vi "Lab Panel V5.22.1.vi"() -> ()   [LabVIEW 2013] (continued)
            n171 = local write "Error USB #0"(w189) -> ()
            n172 = local write "Reset Error"(w189) -> ()
            n173 = local write "Error USB #1"(w189) -> ()
            n174 = local write "Error USB #2"(w189) -> ()
          }
        }
        frame #8 {
          # "get initial temperature values"
          n175 = stacked-sequence {
            frame #0 {
              w196 = T12 {"T1 Live"=20.0, "T1 Neut"=20.0, "T2 Live"=20.0, "T2 Neut"=20.0, "ID"=6.0, "ER"=10.0} ("LAB01 TEMP")
              n176 = local write "LAB deg C"(w196) -> ()
              n177 = global write "Global display 4.vi" "LAB deg C"(w196) -> ()
              n178 = local write "OFF amps"(1.5) -> ()
              n179 = local write "ON amps"(20.0) -> ()
              n180 = local write "VOLTS"(250.0) -> ()
              n181 = local write "PF"(0.5) -> ()
            }
            frame #1 {
              w241 = TRUE
              n182 = local read "Simulate"() -> (w203:bool)
              n183 = local write "Panel #"(0) -> ()
              n184 = case shown="True" w203 {
                frame False {
                }
                frame True {
                  w243 = 20
                  n185 = local write "Ambient Volts"(2.92) -> ()
                  n186 = global write "Global display 3.vi" "Ref deg C"(w243) -> ()
                  n187 = local write "Ref deg C"(w243) -> ()
                }
              }
              n188 = call "sub vi - GET ALL TEMP v7.vi"("LA01-EN"=w241, "simulate"=w203, "LA02-EN"=w241, "LA03-EN"=w241, "LA04-EN"=w241, "LA05-EN"=w241, "Gen Cal Value"=1) -> ("ID"=w202:T24, "LA01 TEMP"=w239:T25, "LA02 TEMP"=w232:T25, "LA03 TEMP"=w225:T25, "LA04 TEMP"=w218:T25, "LA05 TEMP"=w211:T25)  [unwired: 2 in, 1 out]
              n189 = local write "LAB05 TEMP"(w211) -> ()
              n190 = local write "LAB04 TEMP"(w218) -> ()
              n191 = Unbundle(w225) -> ("T1"=w222:dbl, "T2"=w221:dbl, "T3"=w220:dbl, "T4"=w219:dbl)  [unwired: 2 out]
              n192 = Unbundle(w239) -> ("T1"=w237:dbl, "T2"=w236:dbl, "T3"=w235:dbl, "T4"=w234:dbl)  [unwired: 2 out]
              n193 = Unbundle(w232) -> ("T1"=w229:dbl, "T2"=w228:dbl, "T3"=w227:dbl, "T4"=w226:dbl)  [unwired: 2 out]
              n194 = Unbundle(w218) -> ("T1"=w216:dbl, "T2"=w215:dbl, "T3"=w214:dbl, "T4"=w213:dbl)  [unwired: 2 out]
              n195 = Unbundle(w211) -> ("T1"=w209:dbl, "T2"=w208:dbl, "T3"=w207:dbl, "T4"=w206:dbl)  [unwired: 2 out]
              n196 = local write "LAB01 TEMP"(w239) -> ()
              n197 = local write "LAB02 TEMP"(w232) -> ()
              n198 = local write "LAB03 TEMP"(w225) -> ()
              n199 = Unbundle(w202) -> ("id1"=→"LAB01-TP":bool, "id2"=→"LAB02-TP":bool, "id3"=→"LAB03-TP":bool, "id4"=→"LAB04-TP":bool, "id5"=→"LAB05-TP":bool)
              n200 = local read "TEMP LA05"() -> (w210:T9)
              n201 = local read "TEMP LA04"() -> (w217:T9)
              n202 = local read "TEMP LA02"() -> (w231:T9)
              n203 = local read "TEMP LA03"() -> (w224:T9)
              n204 = local read "TEMP LA01"() -> (w238:T9)
              n205 = Bundle(cluster=w224, "TL-1"=w222, "TN-1"=w221, "TL-2"=w220, "TN-2"=w219) -> (w223:T9)  [unwired: 4 in]
              n206 = Bundle(cluster=w238, "TL-1"=w237, "TN-1"=w236, "TL-2"=w235, "TN-2"=w234) -> (w233:T9)  [unwired: 4 in]
              n207 = Bundle(cluster=w231, "TL-1"=w229, "TN-1"=w228, "TL-2"=w227, "TN-2"=w226) -> (w230:T9)  [unwired: 4 in]
              n208 = Bundle(cluster=w217, "TL-1"=w216, "TN-1"=w215, "TL-2"=w214, "TN-2"=w213) -> (w212:T9)  [unwired: 4 in]
              n209 = Bundle(cluster=w210, "TL-1"=w209, "TN-1"=w208, "TL-2"=w207, "TN-2"=w206) -> (w205:T9)  [unwired: 4 in]
              n210 = local write "TEMP LA03"(w223) -> ()
              n211 = local write "TEMP LA01"(w233) -> ()
              n212 = local write "TEMP LA02"(w230) -> ()
              n213 = local write "TEMP LA05"(w205) -> ()
              n214 = local write "TEMP LA04"(w212) -> ()
            }
            frame #2 {
              w252 = 0
              n215 = local read "LAB01 TEMP"() -> (w254:T12)
              n216 = local read "SIG LAB01-2"() -> (w249:T2)
              n217 = Unbundle By Name(w254) -> ("T1 Live"=w247:dbl, "T1 Neut"=w246:dbl, "T2 Live"=w245:dbl, "T2 Neut"=w244:dbl)  [unwired: 2 out]
              n218 = local read "SIG LAB01-1"() -> (w251:T2)
              n219 = local read "TEMP LA01"() -> (w255:T9)
              n220 = Bundle By Name(cluster=w255, "TL-1"=w247, "TN-1"=w246, "TL-2"=w245, "TN-2"=w244, "TL -1COUNT"=w252, "TN-1 COUNT"=w252, "TL-2 COUNT"=w252, "TN-2 COUNT"=w252) -> (w253:T9)
              n221 = Bundle(cluster=w251, "Tmp Live"=w247, "Tmp Neut"=w246) -> (w250:T2)  [unwired: 3 in]
              n222 = Bundle(cluster=w249, "Tmp Live"=w245, "Tmp Neut"=w244) -> (w248:T2)  [unwired: 3 in]
              n223 = local write "SIG LAB01-2"(w248) -> ()
              n224 = local write "SIG LAB01-1"(w250) -> ()
              n225 = local write "TEMP LA01"(w253) -> ()
            }
            frame #3 {
              w264 = 0
              n226 = local read "LAB02 TEMP"() -> (w266:T12)
              n227 = Unbundle By Name(w266) -> ("T1 Live"=w259:dbl, "T1 Neut"=w258:dbl, "T2 Live"=w257:dbl, "T2 Neut"=w256:dbl)  [unwired: 2 out]
              n228 = local read "SIG LAB02-1"() -> (w263:T2)
              n229 = local read "SIG LAB02-2"() -> (w262:T2)
              n230 = local read "TEMP LA02"() -> (w267:T9)
              n231 = Bundle By Name(cluster=w267, "TL-1"=w259, "TN-1"=w258, "TL-2"=w257, "TN-2"=w256, "TL -1COUNT"=w264, "TN-1 COUNT"=w264, "TL-2 COUNT"=w264, "TN-2 COUNT"=w264) -> (w265:T9)
              n232 = Bundle(cluster=w262, "Tmp Live"=w257, "Tmp Neut"=w256) -> (w260:T2)  [unwired: 3 in]
              n233 = Bundle(cluster=w263, "Tmp Live"=w259, "Tmp Neut"=w258) -> (w261:T2)  [unwired: 3 in]
              n234 = local write "TEMP LA02"(w265) -> ()
              n235 = local write "SIG LAB02-1"(w261) -> ()
              n236 = local write "SIG LAB02-2"(w260) -> ()
            }
            frame #4 {
              w276 = 0
              n237 = local read "LAB03 TEMP"() -> (w278:T12)
              n238 = Unbundle By Name(w278) -> ("T1 Live"=w271:dbl, "T1 Neut"=w270:dbl, "T2 Live"=w269:dbl, "T2 Neut"=w268:dbl)  [unwired: 2 out]
              n239 = local read "SIG LAB03-1"() -> (w275:T2)
              n240 = local read "SIG LAB03-2"() -> (w274:T2)
              n241 = local read "TEMP LA03"() -> (w279:T9)
              n242 = Bundle By Name(cluster=w279, "TL-1"=w271, "TN-1"=w270, "TL-2"=w269, "TN-2"=w268, "TL -1COUNT"=w276, "TN-1 COUNT"=w276, "TL-2 COUNT"=w276, "TN-2 COUNT"=w276) -> (w277:T9)
              n243 = Bundle(cluster=w274, "Tmp Live"=w269, "Tmp Neut"=w268) -> (w272:T2)  [unwired: 3 in]
              n244 = Bundle(cluster=w275, "Tmp Live"=w271, "Tmp Neut"=w270) -> (w273:T2)  [unwired: 3 in]
              n245 = local write "TEMP LA03"(w277) -> ()
              n246 = local write "SIG LAB03-2"(w272) -> ()
              n247 = local write "SIG LAB03-1"(w273) -> ()
            }
            frame #5 {
              w288 = 0
              n248 = local read "LAB04 TEMP"() -> (w290:T12)
              n249 = Unbundle By Name(w290) -> ("T1 Live"=w283:dbl, "T1 Neut"=w282:dbl, "T2 Live"=w281:dbl, "T2 Neut"=w280:dbl)  [unwired: 2 out]
              n250 = local read "SIG LAB04-2"() -> (w286:T2)
              n251 = local read "SIG LAB04-1"() -> (w287:T2)
              n252 = local read "TEMP LA04"() -> (w291:T9)
              n253 = Bundle By Name(cluster=w291, "TL-1"=w283, "TN-1"=w282, "TL-2"=w281, "TN-2"=w280, "TL -1COUNT"=w288, "TN-1 COUNT"=w288, "TL-2 COUNT"=w288, "TN-2 COUNT"=w288) -> (w289:T9)
              n254 = Bundle(cluster=w286, "Tmp Live"=w281, "Tmp Neut"=w280) -> (w284:T2)  [unwired: 3 in]
              n255 = Bundle(cluster=w287, "Tmp Live"=w283, "Tmp Neut"=w282) -> (w285:T2)  [unwired: 3 in]
              n256 = local write "SIG LAB04-2"(w284) -> ()
              n257 = local write "TEMP LA04"(w289) -> ()
              n258 = local write "SIG LAB04-1"(w285) -> ()
            }
            frame #6 {
              w300 = 0
              n259 = local read "LAB05 TEMP"() -> (w302:T12)
              n260 = Unbundle By Name(w302) -> ("T1 Live"=w295:dbl, "T1 Neut"=w294:dbl, "T2 Live"=w293:dbl, "T2 Neut"=w292:dbl)  [unwired: 2 out]
              n261 = local read "SIG LAB05-2"() -> (w298:T2)
              n262 = local read "SIG LAB05-1"() -> (w299:T2)
              n263 = local read "TEMP LA05"() -> (w303:T9)
              n264 = Bundle By Name(cluster=w303, "TL-1"=w295, "TN-1"=w294, "TL-2"=w293, "TN-2"=w292, "TL -1COUNT"=w300, "TN-1 COUNT"=w300, "TL-2 COUNT"=w300, "TN-2 COUNT"=w300) -> (w301:T9)
              n265 = Bundle(cluster=w298, "Tmp Live"=w293, "Tmp Neut"=w292) -> (w296:T2)  [unwired: 3 in]
              n266 = Bundle(cluster=w299, "Tmp Live"=w295, "Tmp Neut"=w294) -> (w297:T2)  [unwired: 3 in]
              n267 = local write "SIG LAB05-2"(w296) -> ()
              n268 = local write "SIG LAB05-1"(w297) -> ()
              n269 = local write "TEMP LA05"(w301) -> ()
            }
          }
        }
        frame #9 {
          # "enable front panel, all settings done"
          n270 = property on="Tab Control 2" class="TabCtl (strict)"("DisabledEnum"=T16."Enabled" ("Disabled")) -> ()  [unwired: 2 in, 2 out]
          n271 = property on="Tab Control 2" class="TabCtl (strict)"("Value"=0) -> ()  [unwired: 2 in, 2 out]
        }
        frame #10 {
          n272 = property on="Tab Control 2" class="TabCtl (strict)"("Value"=0) -> ()  [unwired: 2 in, 2 out]
        }
      }
    }
    frame #2 {
      n273 = node-c288("loop  delay(mS)") -> (w309:T18)  [unwired: 3 in]
      n274 = timed-loop {
        timing: w309 -> [_]
        timing-out: [_] -> w308
        i -> [w335]
        stop <- w312 stop-if-true
        n275 = node-c288() -> ()  [unwired: 1 in, 1 out]
        n276 = local read "Resets Done"() -> (w314:dbl)
        n277 = Greater?(x=w314, y=30) -> (0:w310:bool)
        n278 = local read "SELECT LAB05-2"() -> (w315:T3)
        n279 = local read "SELECT LAB05-1"() -> (w316:T3)
        n280 = local read "SELECT LAB04-2"() -> (w317:T3)
        n281 = local read "SELECT LAB03-1"() -> (w320:T3)
        n282 = Or(x=w310, y="stop") -> (x .or. y?=w312:bool)
        n283 = local read "SELECT LAB02-2"() -> (w321:T3)
        n284 = local read "SELECT LAB01-1"() -> (w324:T3)
        n285 = local read "SELECT LAB03-2"() -> (w319:T3)
        n286 = local read "SELECT LAB01-2"() -> (w323:T3)
        n287 = local read "SELECT LAB04-1"() -> (w318:T3)
        n288 = local read "SELECT LAB02-1"() -> (w322:T3)
        n289 = local read "run lab03-2"() -> (w329:bool)
        n290 = local read "run lab04-1"() -> (w328:bool)
        n291 = local read "run lab05-1"() -> (w326:bool)
        n292 = local read "run lab04-2"() -> (w327:bool)
        n293 = local read "run lab05-2"() -> (w325:bool)
        n294 = local read "run lab03-1"() -> (w330:bool)
        n295 = local read "run lab02-2"() -> (w331:bool)
        n296 = local read "run lab02-1"() -> (w332:bool)
        n297 = local read "run lab01-1"() -> (w334:bool)
        n298 = local read "run lab01-2"() -> (w333:bool)
        n299 = global write "Global display 1.vi" "stop disp"(w312) -> ()
        n300 = stacked-sequence {
          seq-local: [_ w401 _ _ _ _ _ _ _ _ _ _ _ _ _ _ _ _ _ _ _ _ _] -> [_ _ _ _ _ w2502 _ _ _ _ _ _ _ _ _ _ _ _ _ _ _ _ _]
          seq-local: [_ w400 _ _ _ _ _ _ _ _ _ _ _ _ _ _ _ _ _ _ _ _ _] -> [_ _ _ _ _ w2501 _ _ _ _ _ _ _ _ _ _ _ _ _ _ _ _ _]
          seq-local: [_ w387 _ _ _ _ _ _ _ _ _ _ _ _ _ _ _ _ _ _ _ _ _] -> [_ _ _ _ _ w2500 _ _ _ _ _ _ _ _ _ _ _ _ _ _ _ _ _]
          seq-local: [_ w386 _ _ _ _ _ _ _ _ _ _ _ _ _ _ _ _ _ _ _ _ _] -> [_ _ _ _ _ w2499 _ _ _ _ _ _ _ _ _ _ _ _ _ _ _ _ _]
          seq-local: [_ w385 _ _ _ _ _ _ _ _ _ _ _ _ _ _ _ _ _ _ _ _ _] -> [_ _ _ _ _ w2498 _ _ _ _ _ _ _ _ _ _ _ _ _ _ _ _ _]
          seq-local: [_ w384 _ _ _ _ _ _ _ _ _ _ _ _ _ _ _ _ _ _ _ _ _] -> [_ _ _ _ _ w2497 _ _ _ _ _ _ _ _ _ _ _ _ _ _ _ _ _]
          seq-local: [_ w383 _ _ _ _ _ _ _ _ _ _ _ _ _ _ _ _ _ _ _ _ _] -> [_ _ _ _ _ w2496 _ _ _ _ _ _ _ _ _ _ _ _ _ _ _ _ _]
          seq-local: [_ w382 _ _ _ _ _ _ _ _ _ _ _ _ _ _ _ _ _ _ _ _ _] -> [_ _ _ _ _ w2495 _ _ _ _ _ _ _ _ _ _ _ _ _ _ _ _ _]
          seq-local: [_ w381 _ _ _ _ _ _ _ _ _ _ _ _ _ _ _ _ _ _ _ _ _] -> [_ _ _ _ _ w2494 _ _ _ _ _ _ _ _ _ _ _ _ _ _ _ _ _]
          seq-local: [_ w380 _ _ _ _ _ _ _ _ _ _ _ _ _ _ _ _ _ _ _ _ _] -> [_ _ _ _ _ w2493 _ _ _ _ _ _ _ _ _ _ _ _ _ _ _ _ _]
          tunnel: w334 -> [_ _ w417 w665 w2092 w2522 w2837 w3324 _ _ _ _ w3893 _ w4850 _ _ w5137 w5440 w5622 _ _ _]
          tunnel: w333 -> [_ _ w416 w663 w2091 w2521 w2838 w3323 _ _ _ _ w3892 _ w4848 _ _ w5136 w5439 w5620 _ _ _]
          tunnel: w332 -> [_ _ w415 w661 w2090 w2520 w2836 w3322 _ _ _ _ w3891 _ w4846 _ _ w5135 w5438 w5619 _ _ _]
          tunnel: w331 -> [_ _ w414 w659 w2089 w2519 w2835 w3321 _ _ _ _ w3890 _ w4844 _ _ w5134 w5437 w5618 _ _ _]
          tunnel: w330 -> [_ _ w413 w657 w2088 w2518 w2834 w3320 _ _ _ _ w3889 _ w4842 _ _ w5133 w5436 w5617 _ _ _]
          tunnel: w329 -> [_ _ w412 w655 w2087 w2517 w2833 w3319 _ _ _ _ w3888 _ w4840 _ _ w5132 w5435 w5616 _ _ _]
          tunnel: w328 -> [_ _ w411 w653 w2086 w2516 w2832 w3318 _ _ _ _ w3887 _ w4838 _ _ w5131 w5434 w5615 _ _ _]
          tunnel: w327 -> [_ _ w410 w651 w2085 w2515 w2831 w3317 _ _ _ _ w3886 _ w4836 _ _ w5130 w5433 w5614 _ _ _]
          tunnel: w326 -> [_ _ w409 w649 w2084 w2514 w2830 w3316 _ _ _ _ w3885 _ w4834 _ _ w5129 w5432 w5613 _ _ _]
          tunnel: w325 -> [_ _ w408 w647 w2083 w2513 w2829 w3315 _ _ _ _ w3884 _ w4832 _ _ w5128 w5431 w5612 _ _ _]
          tunnel: w324 -> [_ _ _ w664 w2082 w2512 _ _ _ _ _ _ _ _ w4852 _ _ _ _ _ w6017 _ _]
          tunnel: w323 -> [_ _ _ w662 w2081 w2511 _ _ _ _ _ _ _ _ w4847 _ _ _ _ _ w6016 _ _]
          tunnel: w322 -> [_ _ _ w660 w2080 w2510 _ _ _ _ _ _ _ _ w4845 _ _ _ _ _ w6015 _ _]
          tunnel: w321 -> [_ _ _ w658 w2079 w2509 _ _ _ _ _ _ _ _ w4843 _ _ _ _ _ w6014 _ _]
          tunnel: w320 -> [_ _ _ w656 w2078 w2508 _ _ _ _ _ _ _ _ w4841 _ _ _ _ _ w6013 _ _]
          tunnel: w319 -> [_ _ _ w654 w2077 w2507 _ _ _ _ _ _ _ _ w4839 _ _ _ _ _ w6012 _ _]
          tunnel: w318 -> [_ _ _ w652 w2076 w2506 _ _ _ _ _ _ _ _ w4837 _ _ _ _ _ w6011 _ _]
          tunnel: w317 -> [_ _ _ w650 w2075 w2505 _ _ _ _ _ _ _ _ w4835 _ _ _ _ _ w6010 _ _]
          tunnel: w316 -> [_ _ _ w648 w2074 w2504 _ _ _ _ _ _ _ _ w4833 _ _ _ _ _ w6009 _ _]
          tunnel: w315 -> [_ _ _ w646 w2073 w2503 _ _ _ _ _ _ _ _ w4831 _ _ _ _ _ w6008 _ _]
          tunnel: w310 -> [_ _ _ _ _ _ _ _ _ _ _ _ _ _ _ _ _ _ _ _ _ _ w6069]
          frame #0 {
            w343 = FALSE
            w348 = 0.5
            # "set up cycle control"
            n301 = local read "jig cycle"() -> (w347:dbl)
            n302 = local read "Amps Fail level"() -> (w341:dbl)
            n303 = local read "Simulate"() -> (w338:bool)
            n304 = Divide(x="JIG ON TIME (S)", y=w348) -> (x/y=→"on loops":dbl)
            n305 = Divide(x="JIG OFF TIME (S)", y=w348) -> (x/y=→"off loops":dbl)
            n306 = Increment(x=w347) -> (x+1=w346:dbl)
            n307 = local write "Simulate IND"(w338) -> ()
            n308 = global write "Global display 3.vi" "Amps Fail"(w341) -> ()
            n309 = local write "TEMP"(w343) -> ()
            n310 = local write "AI"(w343) -> ()
            n311 = local read "Network Directory"() -> (w340:path)
            n312 = local write "jig cycle"(w346) -> ()
            n313 = call "sub vi - check network dir v2.vi"("PATH"=w340) -> ("error"=w339:bool)  [unwired: 10 in]
            n314 = local write "network error"(w339) -> ()
            n315 = global write "Global display 3.vi" "network drive"(w339) -> ()
            n316 = event shown="[1] \"ADMIN\": Value Change" {
              selector: _ -> [_ _]
              dyn-events: _ -> [_ _]
              timeout: 10 -> [_ _]
              event Timeout {
                n317 = event-data() -> ()  [unwired: 1 in, 3 out]
              }
              event "ADMIN": Value Change {
                n318 = event-data() -> ()  [unwired: 1 in, 6 out]
                n319 = stacked-sequence {
                  seq-local: [_ w352 _] -> [_ _ w353]
                  frame #0 {
                    n320 = global write "Global 1.vi" "password"("9949") -> ()
                  }
                  frame #1 {
                    n321 = call "sub vi - password 1.vi"() -> ("RESULT"=w352:bool)  [unwired: 11 in]
                  }
                  frame #2 {
                    w355 = FALSE
                    n322 = property on="Tab Control 2" class="TabCtl (strict)"() -> ("Pages"=w359:refnum<vi>[])  [unwired: 2 in, 2 out]
                    n323 = Select(t=TRUE, s=w353, f=w355) -> (s? t:f=w354:bool)
                    n324 = Index Array(array=w359, index=8) -> (element=w357:refnum<vi>)
                    n325 = property class="Page"(reference=w357, "PageVis"=w354) -> ()  [unwired: 1 in, 2 out]
                    n326 = local write "ADMIN"(w355) -> ()
                  }
                }
              }
            }
          }
          frame #1 {
            w397 = 60.0
            # "convert temperature rise minutes to cycles"
            n327 = local read "SET LAB05-2"() -> (w361:T5)
            n328 = local read "SET LAB05-1"() -> (w363:T5)
            n329 = local read "SET LAB04-2"() -> (w365:T5)
            n330 = local read "SET LAB01-1"() -> (w379:T5)
            n331 = local read "SET LAB01-2"() -> (w377:T5)
            n332 = local read "SET LAB02-2"() -> (w373:T5)
            n333 = local read "SET LAB04-1"() -> (w367:T5)
            n334 = local read "SET LAB03-1"() -> (w371:T5)
            n335 = local read "SET LAB03-2"() -> (w369:T5)
            n336 = local read "SET LAB02-1"() -> (w375:T5)
            n337 = local read "JIG OFF TIME (S)"() -> (w402:dbl)
            n338 = local read "JIG ON TIME (S)"() -> (w403:dbl)
            n339 = Unbundle(w361) -> ("T-RISE mins"=w360:dbl)  [unwired: 4 out]
            n340 = Unbundle(w363) -> ("T-RISE mins"=w362:dbl)  [unwired: 4 out]
            n341 = Unbundle(w379) -> ("T-RISE mins"=w378:dbl)  [unwired: 4 out]
            n342 = Unbundle(w365) -> ("T-RISE mins"=w364:dbl)  [unwired: 4 out]
            n343 = Unbundle(w377) -> ("T-RISE mins"=w376:dbl)  [unwired: 4 out]
            n344 = Unbundle(w375) -> ("T-RISE mins"=w374:dbl)  [unwired: 4 out]
            n345 = Unbundle(w367) -> ("T-RISE mins"=w366:dbl)  [unwired: 4 out]
            n346 = Unbundle(w373) -> ("T-RISE mins"=w372:dbl)  [unwired: 4 out]
            n347 = Unbundle(w369) -> ("T-RISE mins"=w368:dbl)  [unwired: 4 out]
            n348 = Unbundle(w371) -> ("T-RISE mins"=w370:dbl)  [unwired: 4 out]
            n349 = Add(x=w403, y=w402) -> (x+y=w396:dbl)
            n350 = Multiply(x=w397, y=w368) -> (x*y=w392:dbl)
            n351 = Multiply(x=w397, y=w366) -> (x*y=w391:dbl)
            n352 = Multiply(x=w397, y=w364) -> (x*y=w390:dbl)
            n353 = Multiply(x=w397, y=w362) -> (x*y=w389:dbl)
            n354 = Multiply(x=w397, y=w360) -> (x*y=w388:dbl)
            n355 = Multiply(x=w397, y=w376) -> (x*y=w398:dbl)
            n356 = Multiply(x=w397, y=w370) -> (x*y=w393:dbl)
            n357 = Multiply(x=w397, y=w378) -> (x*y=w399:dbl)
            n358 = Multiply(x=w397, y=w374) -> (x*y=w395:dbl)
            n359 = Multiply(x=w397, y=w372) -> (x*y=w394:dbl)
            n360 = Divide(x=w389, y=w396) -> (x/y=w381:dbl)
            n361 = Divide(x=w390, y=w396) -> (x/y=w382:dbl)
            n362 = Divide(x=w391, y=w396) -> (x/y=w383:dbl)
            n363 = Divide(x=w388, y=w396) -> (x/y=w380:dbl)
            n364 = Divide(x=w393, y=w396) -> (x/y=w385:dbl)
            n365 = Divide(x=w399, y=w396) -> (x/y=w401:dbl)
            n366 = Divide(x=w398, y=w396) -> (x/y=w400:dbl)
            n367 = Divide(x=w395, y=w396) -> (x/y=w387:dbl)
            n368 = Divide(x=w394, y=w396) -> (x/y=w386:dbl)
            n369 = Divide(x=w392, y=w396) -> (x/y=w384:dbl)
          }
          frame #2 {
            # "control cycle loops"
            n370 = local read "JIG OFF TIME (S)"() -> (w406:dbl)
            n371 = local read "JIG ON TIME (S)"() -> (w405:dbl)
            n372 = local read "jig cycle"() -> (w419:dbl)
            n373 = local read "on loops"() -> (w421:dbl)
            n374 = local read "off loops"() -> (w420:dbl)
            n375 = Add(x=w406, y=w405) -> (x+y=w404:dbl)
            n376 = Add(x=w421, y=w420) -> (x+y=w407:dbl)
            n377 = Greater Or Equal?(x=w419, y=w407) -> (x >= y?=w418:bool)
            n378 = case shown="True" w418 {
              tunnel: w417 -> [_ w455]
              tunnel: w416 -> [_ w454]
              tunnel: w415 -> [_ w453]
              tunnel: w414 -> [_ w452]
              tunnel: w413 -> [_ w451]
              tunnel: w412 -> [_ w450]
              tunnel: w411 -> [_ w449]
              tunnel: w410 -> [_ w448]
              tunnel: w409 -> [_ w447]
              tunnel: w408 -> [_ w446]
              tunnel: w404 -> [_ w445]
              frame False {
              }
              frame True {
                # "increment cycle value and convert cycles to minutes for temp rise"
                n379 = stacked-sequence {
                  frame #0 {
                    n380 = local read "Panel #"() -> (w458:dbl)
                    n381 = Increment(x=w458) -> (x+1=w457:dbl)
                    n382 = local write "Panel #"(w457) -> ()
                  }
                  frame #1 {
                    n383 = local read "Panel #"() -> (w459:dbl)
                    n384 = Greater?(x=w459, y=5) -> (0:w461:bool)
                    n385 = case shown="True" w461 {
                      frame False {
                      }
                      frame True {
                        n386 = local write "Panel #"(1) -> ()
                      }
                    }
                  }
                }
                n387 = local read "JIG RELAY CYCLES"() -> (w444:T8)
                n388 = local read "Panel #"() -> (→"Tp Ut":dbl)
                n389 = Unbundle By Name(w444) -> ("LAB01-1"=w442:dbl, "LAB01-2"=w440:dbl, "LAB02-1"=w438:dbl, "LAB02-2"=w436:dbl, "LAB03-1"=w434:dbl, "LAB03-2"=w432:dbl, "LAB04-1"=w430:dbl, "LAB04-2"=w428:dbl, "LAB05-1"=w426:dbl, "LAB05-2"=w424:dbl)
                n390 = stacked-sequence {
                  tunnel: w455 -> [w473 _ _ _ _ _ _ _ _ _]
                  tunnel: w454 -> [_ w490 _ _ _ _ _ _ _ _]
                  tunnel: w453 -> [_ _ w507 _ _ _ _ _ _ _]
                  tunnel: w452 -> [_ _ _ w524 _ _ _ _ _ _]
                  tunnel: w451 -> [_ _ _ _ w541 _ _ _ _ _]
                  tunnel: w450 -> [_ _ _ _ _ w558 _ _ _ _]
                  tunnel: w449 -> [_ _ _ _ _ _ w575 _ _ _]
                  tunnel: w448 -> [_ _ _ _ _ _ _ w592 _ _]
                  tunnel: w447 -> [_ _ _ _ _ _ _ _ w609 _]
                  tunnel: w446 -> [_ _ _ _ _ _ _ _ _ w626]
                  tunnel: w445 -> [w470 w487 w504 w521 w538 w555 w572 w589 w606 w623]
                  tunnel: w442 -> [w464 _ _ _ _ _ _ _ _ _]
                  tunnel: [w463 _ _ _ _ _ _ _ _ _] -> w441
                  tunnel: w440 -> [_ w481 _ _ _ _ _ _ _ _]
                  tunnel: [_ w480 _ _ _ _ _ _ _ _] -> w439
                  tunnel: w438 -> [_ _ w498 _ _ _ _ _ _ _]
                  tunnel: [_ _ w497 _ _ _ _ _ _ _] -> w437
                  tunnel: w436 -> [_ _ _ w515 _ _ _ _ _ _]
                  tunnel: [_ _ _ w514 _ _ _ _ _ _] -> w435
                  tunnel: w434 -> [_ _ _ _ w532 _ _ _ _ _]
                  tunnel: [_ _ _ _ w531 _ _ _ _ _] -> w433
                  tunnel: w432 -> [_ _ _ _ _ w549 _ _ _ _]
                  tunnel: [_ _ _ _ _ w548 _ _ _ _] -> w431
                  tunnel: w430 -> [_ _ _ _ _ _ w566 _ _ _]
                  tunnel: [_ _ _ _ _ _ w565 _ _ _] -> w429
                  tunnel: w428 -> [_ _ _ _ _ _ _ w583 _ _]
                  tunnel: [_ _ _ _ _ _ _ w582 _ _] -> w427
                  tunnel: w426 -> [_ _ _ _ _ _ _ _ w600 _]
                  tunnel: [_ _ _ _ _ _ _ _ w599 _] -> w425
                  tunnel: w424 -> [_ _ _ _ _ _ _ _ _ w617]
                  tunnel: [_ _ _ _ _ _ _ _ _ w616] -> w423
                  frame #0 {
                    n391 = local read "DISP LAB01-1"() -> (w468:T4)
                    n392 = Unbundle(w468) -> ("CYCLE"=w469:dbl)  [unwired: 2 out]
                    n393 = case shown="True" w473 {
                      tunnel: w469 -> [w475 w479]
                      tunnel: [w475 w478] -> w467
                      tunnel: w464 -> [w474 w477]
                      tunnel: [w474 w476] -> w463
                      frame False {
                      }
                      frame True {
                        n394 = Increment(x=w477) -> (x+1=w476:dbl)
                        n395 = Increment(x=w479) -> (x+1=w478:dbl)
                      }
                    }
                    n396 = Multiply(x=w467, y=w470) -> (x*y=w471:dbl)
                    n397 = Divide(x=w471, y=60.0) -> (x/y=w466:dbl)
                    n398 = Bundle(cluster=w468, "CYCLE"=w467, "MINS"=w466) -> (w465:T4)  [unwired: 1 in]
                    n399 = local write "DISP LAB01-1"(w465) -> ()
                  }
                  frame #1 {
                    n400 = local read "DISP LAB01-2"() -> (w485:T4)
                    n401 = Unbundle(w485) -> ("CYCLE"=w486:dbl)  [unwired: 2 out]
                    n402 = case shown="True" w490 {
                      tunnel: w486 -> [w492 w496]
                      tunnel: [w492 w495] -> w483
                      tunnel: w481 -> [w491 w494]
                      tunnel: [w491 w493] -> w480
                      frame False {
                      }
                      frame True {
                        n403 = Increment(x=w494) -> (x+1=w493:dbl)
                        n404 = Increment(x=w496) -> (x+1=w495:dbl)
                      }
                    }
                    n405 = Multiply(x=w483, y=w487) -> (x*y=w488:dbl)
                    n406 = Divide(x=w488, y=60.0) -> (x/y=w482:dbl)
                    n407 = Bundle(cluster=w485, "CYCLE"=w483, "MINS"=w482) -> (w484:T4)  [unwired: 1 in]
                    n408 = local write "DISP LAB01-2"(w484) -> ()
                  }
                  frame #2 {
                    n409 = local read "DISP LAB02-1"() -> (w502:T4)
                    n410 = Unbundle(w502) -> ("CYCLE"=w503:dbl)  [unwired: 2 out]
                    n411 = case shown="True" w507 {
                      tunnel: [w509 w513] -> w500
                      tunnel: w503 -> [w509 w512]
                      tunnel: w498 -> [w508 w511]
                      tunnel: [w508 w510] -> w497
                      frame False {
                      }
                      frame True {
                        n412 = Increment(x=w511) -> (x+1=w510:dbl)
                        n413 = Increment(x=w512) -> (x+1=w513:dbl)
                      }
                    }
                    n414 = Multiply(x=w500, y=w504) -> (x*y=w505:dbl)
                    n415 = Divide(x=w505, y=60.0) -> (x/y=w499:dbl)
                    n416 = Bundle(cluster=w502, "CYCLE"=w500, "MINS"=w499) -> (w501:T4)  [unwired: 1 in]
                    n417 = local write "DISP LAB02-1"(w501) -> ()
                  }
                  frame #3 {
                    n418 = local read "DISP LAB02-2"() -> (w519:T4)
                    n419 = Unbundle(w519) -> ("CYCLE"=w520:dbl)  [unwired: 2 out]
                    n420 = case shown="True" w524 {
                      tunnel: [w526 w530] -> w518
                      tunnel: w520 -> [w526 w529]
                      tunnel: w515 -> [w525 w528]
                      tunnel: [w525 w527] -> w514
                      frame False {
                      }
                      frame True {
                        n421 = Increment(x=w528) -> (x+1=w527:dbl)
                        n422 = Increment(x=w529) -> (x+1=w530:dbl)
                      }
                    }
                    n423 = Multiply(x=w518, y=w521) -> (x*y=w522:dbl)
                    n424 = Divide(x=w522, y=60.0) -> (x/y=w517:dbl)
                    n425 = Bundle(cluster=w519, "CYCLE"=w518, "MINS"=w517) -> (w516:T4)  [unwired: 1 in]
                    n426 = local write "DISP LAB02-2"(w516) -> ()
                  }
                  frame #4 {
                    n427 = local read "DISP LAB03-1"() -> (w536:T4)
                    n428 = Unbundle(w536) -> ("CYCLE"=w537:dbl)  [unwired: 2 out]
                    n429 = case shown="True" w541 {
                      tunnel: [w543 w547] -> w533
                      tunnel: w537 -> [w543 w546]
                      tunnel: w532 -> [w542 w545]
                      tunnel: [w542 w544] -> w531
                      frame False {
                      }
                      frame True {
                        n430 = Increment(x=w545) -> (x+1=w544:dbl)
                        n431 = Increment(x=w546) -> (x+1=w547:dbl)
                      }
                    }
                    n432 = Multiply(x=w533, y=w538) -> (x*y=w539:dbl)
                    n433 = Divide(x=w539, y=60.0) -> (x/y=w534:dbl)
                    n434 = Bundle(cluster=w536, "CYCLE"=w533, "MINS"=w534) -> (w535:T4)  [unwired: 1 in]
                    n435 = local write "DISP LAB03-1"(w535) -> ()
                  }
                  frame #5 {
                    n436 = local read "DISP LAB03-2"() -> (w553:T4)
                    n437 = Unbundle(w553) -> ("CYCLE"=w554:dbl)  [unwired: 2 out]
                    n438 = case shown="True" w558 {
                      tunnel: [w560 w564] -> w552
                      tunnel: w554 -> [w560 w563]
                      tunnel: w549 -> [w559 w562]
                      tunnel: [w559 w561] -> w548
                      frame False {
                      }
                      frame True {
                        n439 = Increment(x=w562) -> (x+1=w561:dbl)
                        n440 = Increment(x=w563) -> (x+1=w564:dbl)
                      }
                    }
                    n441 = Multiply(x=w552, y=w555) -> (x*y=w556:dbl)
                    n442 = Divide(x=w556, y=60.0) -> (x/y=w551:dbl)
                    n443 = Bundle(cluster=w553, "CYCLE"=w552, "MINS"=w551) -> (w550:T4)  [unwired: 1 in]
                    n444 = local write "DISP LAB03-2"(w550) -> ()
                  }
                  frame #6 {
                    n445 = local read "DISP LAB04-1"() -> (w570:T4)
                    n446 = Unbundle(w570) -> ("CYCLE"=w571:dbl)  [unwired: 2 out]
                    n447 = case shown="True" w575 {
                      tunnel: [w577 w581] -> w568
                      tunnel: w571 -> [w577 w580]
                      tunnel: w566 -> [w576 w579]
                      tunnel: [w576 w578] -> w565
                      frame False {
                      }
                      frame True {
                        n448 = Increment(x=w579) -> (x+1=w578:dbl)
                        n449 = Increment(x=w580) -> (x+1=w581:dbl)
                      }
                    }
                    n450 = Multiply(x=w568, y=w572) -> (x*y=w573:dbl)
                    n451 = Divide(x=w573, y=60.0) -> (x/y=w567:dbl)
                    n452 = Bundle(cluster=w570, "CYCLE"=w568, "MINS"=w567) -> (w569:T4)  [unwired: 1 in]
                    n453 = local write "DISP LAB04-1"(w569) -> ()
                  }
                  frame #7 {
                    n454 = local read "DISP LAB04-2"() -> (w587:T4)
                    n455 = Unbundle(w587) -> ("CYCLE"=w588:dbl)  [unwired: 2 out]
                    n456 = case shown="True" w592 {
                      tunnel: [w594 w598] -> w585
                      tunnel: w588 -> [w594 w597]
                      tunnel: w583 -> [w593 w596]
                      tunnel: [w593 w595] -> w582
                      frame False {
                      }
                      frame True {
                        n457 = Increment(x=w596) -> (x+1=w595:dbl)
                        n458 = Increment(x=w597) -> (x+1=w598:dbl)
                      }
                    }
                    n459 = Multiply(x=w585, y=w589) -> (x*y=w591:dbl)
                    n460 = Divide(x=w591, y=60.0) -> (x/y=w584:dbl)
                    n461 = Bundle(cluster=w587, "CYCLE"=w585, "MINS"=w584) -> (w586:T4)  [unwired: 1 in]
                    n462 = local write "DISP LAB04-2"(w586) -> ()
                  }
                  frame #8 {
                    n463 = local read "DISP LAB05-1"() -> (w604:T4)
                    n464 = Unbundle(w604) -> ("CYCLE"=w605:dbl)  [unwired: 2 out]
                    n465 = case shown="True" w609 {
                      tunnel: [w611 w615] -> w602
                      tunnel: w605 -> [w611 w614]
                      tunnel: w600 -> [w610 w613]
                      tunnel: [w610 w612] -> w599
                      frame False {
                      }
                      frame True {
                        n466 = Increment(x=w613) -> (x+1=w612:dbl)
                        n467 = Increment(x=w614) -> (x+1=w615:dbl)
                      }
                    }
                    n468 = Multiply(x=w602, y=w606) -> (x*y=w607:dbl)
                    n469 = Divide(x=w607, y=60.0) -> (x/y=w601:dbl)
                    n470 = Bundle(cluster=w604, "CYCLE"=w602, "MINS"=w601) -> (w603:T4)  [unwired: 1 in]
                    n471 = local write "DISP LAB05-1"(w603) -> ()
                  }
                  frame #9 {
                    n472 = local read "DISP LAB05-2"() -> (w622:T4)
                    n473 = Unbundle(w622) -> ("CYCLE"=w621:dbl)  [unwired: 2 out]
                    n474 = case shown="True" w626 {
                      tunnel: [w628 w632] -> w620
                      tunnel: w621 -> [w628 w631]
                      tunnel: w617 -> [w627 w630]
                      tunnel: [w627 w629] -> w616
                      frame False {
                      }
                      frame True {
                        n475 = Increment(x=w630) -> (x+1=w629:dbl)
                        n476 = Increment(x=w631) -> (x+1=w632:dbl)
                      }
                    }
                    n477 = Multiply(x=w620, y=w623) -> (x*y=w624:dbl)
                    n478 = Divide(x=w624, y=60.0) -> (x/y=w619:dbl)
                    n479 = Bundle(cluster=w622, "CYCLE"=w620, "MINS"=w619) -> (w618:T4)  [unwired: 1 in]
                    n480 = local write "DISP LAB05-2"(w618) -> ()
                  }
                }
                n481 = local write "jig cycle"(0) -> ()
                n482 = Bundle By Name(cluster=w444, "LAB01-1"=w441, "LAB01-2"=w439, "LAB02-1"=w437, "LAB02-2"=w435, "LAB03-1"=w433, "LAB03-2"=w431, "LAB04-1"=w429, "LAB04-2"=w427, "LAB05-1"=w425, "LAB05-2"=w423) -> (w443:T8)
                n483 = local write "JIG RELAY CYCLES"(w443) -> ()
              }
            }
          }
          frame #3 {
            # "START & STOP test RUN switch change, start test if true and stop test if false"
            n484 = Get Date/Time In Seconds() -> (seconds since 1Jan1904=w644:timestamp)
            n485 = local read "C drive data root dir"() -> (w637:path)
            n486 = Format Date/Time String(time format string (%c)="%b\\%a%d", seconds (now)=w644) -> (date/time string=w668:string)  [unwired: 1 in]
            n487 = Format Date/Time String(time format string (%c)="%H%M", seconds (now)=w644) -> (date/time string=w666:string)  [unwired: 1 in]
            n488 = Format Date/Time String(time format string (%c)="LabPanel%Y", seconds (now)=w644) -> (date/time string=w643:string)  [unwired: 1 in]
            n489 = Path To String(path=w637) -> (string=w640:string)
            n490 = global write "Global 1.vi" "C drive root path"(w637) -> ()
            n491 = local read "Ref deg C"() -> (w633:dbl)
            n492 = Concatenate Strings(w640, "\\") -> (w638:string)
            n493 = event shown="[1] \"RUN LAB01-1\": Value Change" {
              selector: _ -> [_ _ _ _ _ _ _ _ _ _ _]
              dyn-events: _ -> [_ _ _ _ _ _ _ _ _ _ _]
              timeout: 10 -> [_ _ _ _ _ _ _ _ _ _ _]
              tunnel: w638 -> [_ w681 w821 w962 w1102 w1242 w1382 w1522 w1662 w1802 w1943]
              tunnel: w668 -> [_ w680 w820 w961 w1101 w1241 w1381 w1521 w1661 w1801 w1942]
              tunnel: w666 -> [_ w678 w819 w960 w1100 w1240 w1380 w1520 w1660 w1800 w1941]
              tunnel: w664 -> [_ w679 _ _ _ _ _ _ _ _ _]
              tunnel: w665 -> [_ _ _ _ _ _ _ _ _ _ _]
              tunnel: w663 -> [_ _ _ _ _ _ _ _ _ _ _]
              tunnel: w662 -> [_ _ w818 _ _ _ _ _ _ _ _]
              tunnel: w661 -> [_ _ _ _ _ _ _ _ _ _ _]
              tunnel: w660 -> [_ _ _ w959 _ _ _ _ _ _ _]
              tunnel: w659 -> [_ _ _ _ _ _ _ _ _ _ _]
              tunnel: w658 -> [_ _ _ _ w1099 _ _ _ _ _ _]
              tunnel: w657 -> [_ _ _ _ _ _ _ _ _ _ _]
              tunnel: w656 -> [_ _ _ _ _ w1239 _ _ _ _ _]
              tunnel: w655 -> [_ _ _ _ _ _ _ _ _ _ _]
              tunnel: w654 -> [_ _ _ _ _ _ w1379 _ _ _ _]
              tunnel: w653 -> [_ _ _ _ _ _ _ _ _ _ _]
              tunnel: w652 -> [_ _ _ _ _ _ _ w1519 _ _ _]
              tunnel: w651 -> [_ _ _ _ _ _ _ _ _ _ _]
              tunnel: w650 -> [_ _ _ _ _ _ _ _ w1659 _ _]
              tunnel: w649 -> [_ _ _ _ _ _ _ _ _ _ _]
              tunnel: w648 -> [_ _ _ _ _ _ _ _ _ w1799 _]
              tunnel: w647 -> [_ _ _ _ _ _ _ _ _ _ _]
              tunnel: w646 -> [_ _ _ _ _ _ _ _ _ _ w1940]
              tunnel: w643 -> [_ w677 w817 w958 w1098 w1238 w1378 w1518 w1658 w1798 w1939]
              tunnel: [_ w676 w816 w957 w1097 w1237 w1377 w1517 w1657 w1797 w1938] -> w641
              tunnel: "RESET CYCLES TO ZERO?" -> [_ w675 w814 w955 w1095 w1235 w1375 w1515 w1655 w1795 w1936]
              tunnel: "YES" -> [_ w674 w813 w954 w1094 w1234 w1374 w1514 w1654 w1794 w1935]
              tunnel: "NO" -> [_ w673 w812 w953 w1093 w1233 w1373 w1513 w1653 w1793 w1934]
              tunnel: w633 -> [_ w670 w811 w951 w1092 w1232 w1372 w1512 w1652 w1792 w1932]
              event Timeout {
                n494 = event-data() -> ()  [unwired: 1 in, 3 out]
              }
              event "RUN LAB01-1": Value Change {
                n495 = event-data() -> ("NewVal"=w671:bool)  [unwired: 1 in, 5 out]
                n496 = local read "SIG LAB01-1"() -> (w672:T2)
                n497 = local write "run lab01-1"(w671) -> ()
                n498 = case shown="True" w671 {
                  tunnel: w681 -> [_ w719]
                  tunnel: w680 -> [_ w718]
                  tunnel: w679 -> [w683 w717]
                  tunnel: w678 -> [_ w716]
                  tunnel: w677 -> [_ w715]
                  tunnel: [w682 w714] -> w676
                  tunnel: w675 -> [_ w713]
                  tunnel: w674 -> [_ w712]
                  tunnel: w673 -> [_ w711]
                  tunnel: w672 -> [_ w710]
                  tunnel: w670 -> [_ w709]
                  frame False {
                    # "stop test"
                    n499 = stacked-sequence {
                      tunnel: w683 -> [_ w695 _]
                      tunnel: [_ w687 _] -> w682
                      frame #0 {
                        n500 = local read "DISP LAB01-1"() -> (w686:T4)
                        n501 = Bundle(cluster=w686, "STATUS"="STOP") -> (w684:T4)  [unwired: 2 in]
                        n502 = local write "DISP LAB01-1"(w684) -> ()
                      }
                      frame #1 {
                        n503 = local read "DISP LAB01-1"() -> (w694:T4)
                        n504 = Unbundle(w694) -> ("CYCLE"=w692:dbl, "MINS"=w693:dbl)  [unwired: 1 out]
                        n505 = case shown="\"CYCLE TEST\"" w695 {
                          tunnel: w693 -> [_ _ w702]
                          tunnel: w692 -> [w700 w701 _]
                          tunnel: [w700 w701 w702] -> w691
                          frame "CHART TEST", Default {
                          }
                          frame "CYCLE TEST" {
                          }
                          frame "T-RISE TEST" {
                          }
                        }
                        n506 = local read "TDMS LAB01-1"() -> (w699:refnum<k34>)
                        n507 = Build Array("STOPPED") -> (w696:string[])
                        n508 = Build Array(w691) -> (w690:dbl[])
                        n509 = TDMS Write(0:w699, 5:"TEST RESULT", 7:w696, 9:w690) -> (4:w688:refnum<k34>, 15:w689:errorcluster)  [unwired: 2 in, 2 out]
                        n510 = TDMS Close(8:w689, 11:w688) -> (0:w687:errorcluster)  [unwired: 1 out]
                      }
                      frame #2 {
                        n511 = stacked-sequence {
                          tunnel: "LAB01-1" -> [w705 w707]
                          frame #0 {
                            n512 = call "sub vi - defrag tdms v1.vi"("panel id"=w705) -> ("error out"=w704:errorcluster)  [unwired: 10 in]
                            n513 = local write "data file error"(w704) -> ()
                          }
                          frame #1 {
                            n514 = call "Save data file (stop) v3.vi"("panel id"=w707) -> ("network file save error"=w706:errorcluster)  [unwired: 9 in, 1 out]
                            n515 = local write "RESULT LAB01-1"(FALSE) -> ()
                            n516 = local write "data file error"(w706) -> ()
                          }
                        }
                      }
                    }
                  }
                  frame True {
                    n517 = stacked-sequence {
                      seq-local: [w721 _] -> [_ w725]
                      tunnel: w719 -> [_ w735]
                      tunnel: w718 -> [_ w734]
                      tunnel: w717 -> [_ w733]
                      tunnel: w716 -> [_ w732]
                      tunnel: w715 -> [_ w731]
                      tunnel: [_ w730] -> w714
                      tunnel: w713 -> [_ w729]
                      tunnel: w712 -> [_ w728]
                      tunnel: w711 -> [_ w727]
                      tunnel: w710 -> [w723 w726]
                      tunnel: w709 -> [_ w724]
                      frame #0 {
                        n518 = Unbundle(w723) -> ("AMPS"=w722:dbl)  [unwired: 4 out]
                        n519 = call "Check For Amps on v1.vi"("ID"="LAB01-1", "amps"=w722) -> ("amps"=w721:bool)  [unwired: 9 in]
                      }
                      frame #1 {
                        n520 = case shown="True" w725 {
                          tunnel: w735 -> [_ w748]
                          tunnel: w734 -> [_ w747]
                          tunnel: w733 -> [_ w746]
                          tunnel: w732 -> [_ w745]
                          tunnel: w731 -> [_ w744]
                          tunnel: [errorcluster {"status"=FALSE, "code"=0, "source"=""} ("error out") w743] -> w730
                          tunnel: w729 -> [_ w742]
                          tunnel: w728 -> [_ w741]
                          tunnel: w727 -> [_ w740]
                          tunnel: w726 -> [_ w739]
                          tunnel: w724 -> [_ w738]
                          frame False {
                            w736 = FALSE
                            n521 = local write "RUN LAB01-1"(w736) -> ()
                            n522 = local write "run lab01-1"(w736) -> ()
                          }
                          frame True {
                            n523 = stacked-sequence {
                              seq-local: [w749 _ _ _ _] -> [_ w770 _ _ _]
                              tunnel: w748 -> [w754 _ _ _ _]
                              tunnel: w747 -> [w750 _ _ _ _]
                              tunnel: w746 -> [w764 _ _ _ _]
                              tunnel: w745 -> [w757 _ _ _ _]
                              tunnel: w744 -> [w752 _ _ _ _]
                              tunnel: [_ w771 _ _ _] -> w743
                              tunnel: w742 -> [_ _ _ w792 _]
                              tunnel: w741 -> [_ _ _ w802 _]
                              tunnel: w740 -> [_ _ _ w801 _]
                              tunnel: w739 -> [_ _ _ _ _]
                              tunnel: w738 -> [_ _ _ _ w808]
                              frame #0 {
                                w751 = "\\"
                                n524 = case shown="\"CHART TEST\", Default" w764 {
                                tunnel: ["L01-1-CHART TEST-" "L01-1-CYCLE TEST-" "L01-1-T-RISE TEST-"] -> w760
                                frame "CHART TEST", Default {
                                }
                                frame "CYCLE TEST" {
                                }
                                frame "T-RISE TEST" {
                                }
                                }
                                n525 = local read "SET LAB01-1"() -> (w759:T5)
                                n526 = Unbundle(w759) -> ("DESCRIPTION"=w758:string)  [unwired: 4 out]
                                n527 = Concatenate Strings(w754, "\\", w752, w751, w750, w751) -> (w761:string)
                                n528 = String To Path(string=w761) -> (path=w763:path)
                                n529 = Concatenate Strings(w761, w760, w758, "-", w757, ".tdms") -> (w749:string)
                                n530 = Create Folder(path (use dialog)=w763) -> (error out=w762:errorcluster)  [unwired: 2 in, 2 out]
                                n531 = call <vilib>:"Clear Errors.vi"("error in (no error)"=w762) -> ()  [unwired: 6 in, 1 out]
                                n532 = global write "Global 1.vi" "LAB01-1 FILE"(w749) -> ()
                              }
                              frame #1 {
                                (unwired) FALSE
                                n533 = String To Path(string=w770) -> (path=w768:path)
                                n534 = TDMS Open(6:FALSE, 10:T21."create or replace" ("operation (0:open)"), 11:w768) -> (0:w771:errorcluster, 3:→"TDMS LAB01-1":refnum<k34>)  [unwired: 4 in]
                              }
                              frame #2 {
                                n535 = local read "TDMS LAB01-1"() -> (w790:refnum<k34>)
                                n536 = local read "SET LAB01-1"() -> (w779:T5)
                                n537 = Build Array("Testers Name", "Description", "Set Test Cycles", "T-Rise minutes", "T-Rise Deg C") -> (w780:string[])
                                n538 = Unbundle(w779) -> ("NAME"=w778:string, "DESCRIPTION"=w777:string, "CYCLES"=w776:dbl, "T-RISE mins"=w775:dbl, "T-RISE deg C"=w774:dbl)
                                n539 = Number To Decimal String(number=w776) -> (decimal integer string=w789:string)  [unwired: 1 in]
                                n540 = Number To Decimal String(number=w775) -> (decimal integer string=w788:string)  [unwired: 1 in]
                                n541 = Number To Decimal String(number=w774) -> (decimal integer string=w787:string)  [unwired: 1 in]
                                n542 = Build Array(w778, w777, w789, w788, w787) -> (w786:string[])
                                n543 = TDMS Set Properties(5:w786, 7:w780, 11:w790) -> ()  [unwired: 3 in, 4 out]
                              }
                              frame #3 {
                                n544 = local read "DISP LAB01-1"() -> (w800:T4)
                                n545 = Concatenate Strings("LAB01-1  ", w792) -> (w791:string)
                                n546 = Two Button Dialog(message=w791, 1:w801, 2:w802) -> (T button?=w794:bool)
                                n547 = case shown="True" w794 {
                                tunnel: w800 -> [w805 w806]
                                tunnel: [w805 w806] -> w799
                                tunnel: [w804 w807] -> w798
                                tunnel: [w803 w807] -> w797
                                frame False {
                                n548 = Unbundle(w805) -> ("CYCLE"=w804:dbl, "MINS"=w803:dbl)  [unwired: 1 out]
                                }
                                frame True {
                                w807 = 0.0
                                }
                                }
                                n549 = Bundle(cluster=w799, "CYCLE"=w798, "MINS"=w797, "STATUS"="RUN") -> (w796:T4)
                                n550 = local write "DISP LAB01-1"(w796) -> ()
                              }
                              frame #4 {
                                n551 = local read "TEMP START LAB01-1"() -> (w810:cluster{"TL":dbl, "TN":dbl})
                                n552 = Bundle(cluster=w810, "TL"=w808, "TN"=w808) -> (w809:cluster{"TL":dbl, "TN":dbl})
                                n553 = local write "TEMP START LAB01-1"(w809) -> ()
                              }
                            }
                          }
                        }
                      }
                    }
                  }
                }
              }
              event "RUN LAB01-2": Value Change {
                n554 = event-data() -> ("NewVal"=w815:bool)  [unwired: 1 in, 5 out]
                n555 = local write "run lab01-2"(w815) -> ()
                n556 = case shown="True" w815 {
                  tunnel: w821 -> [_ w859]
                  tunnel: w820 -> [_ w858]
                  tunnel: w818 -> [w823 w857]
                  tunnel: w819 -> [_ w856]
                  tunnel: w817 -> [_ w855]
                  tunnel: [w822 w854] -> w816
                  tunnel: w814 -> [_ w853]
                  tunnel: w813 -> [_ w852]
                  tunnel: w812 -> [_ w851]
                  tunnel: w811 -> [_ w849]
                  frame False {
                    # "stop test"
                    n557 = stacked-sequence {
                      tunnel: w823 -> [w832 _]
                      tunnel: [w824 _] -> w822
                      frame #0 {
                        n558 = local read "DISP LAB01-2"() -> (w831:T4)
                        n559 = Unbundle(w831) -> ("CYCLE"=w829:dbl, "MINS"=w830:dbl)  [unwired: 1 out]
                        n560 = case shown="\"CHART TEST\", Default" w832 {
                          tunnel: w830 -> [_ _ w839]
                          tunnel: w829 -> [w837 w838 _]
                          tunnel: [w837 w838 w839] -> w828
                          frame "CHART TEST", Default {
                          }
                          frame "CYCLE TEST" {
                          }
                          frame "T-RISE TEST" {
                          }
                        }
                        n561 = local read "TDMS LAB01-2"() -> (w836:refnum<k34>)
                        n562 = Build Array("STOPPED") -> (w833:string[])
                        n563 = Build Array(w828) -> (w827:dbl[])
                        n564 = TDMS Write(0:w836, 5:"TEST RESULT", 7:w833, 9:w827) -> (4:w825:refnum<k34>, 15:w826:errorcluster)  [unwired: 2 in, 2 out]
                        n565 = TDMS Close(8:w826, 11:w825) -> (0:w824:errorcluster)  [unwired: 1 out]
                      }
